vi "Floor_Negative.vi"(8 "Cutoff U8":u8, 10 "Baseline U8":u8, 11 "Input Value":u8) -> (0 "Over?":bool, 3 "Output Value":u8)   [LabVIEW 2012]
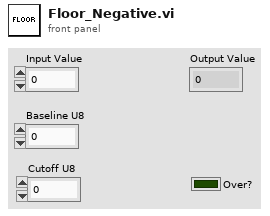
[diagram p1: front panel]
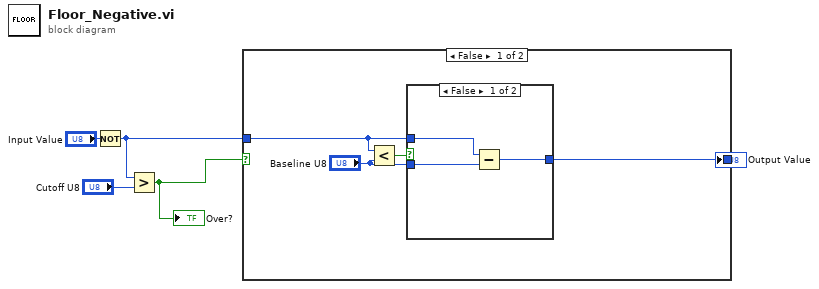
[diagram p0: block diagram]
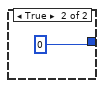
[diagram p2: hidden frame]
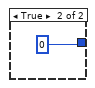
[diagram p3: hidden frame]
diagram:
  n1 = Not(x="Input Value") -> (.not. x?=w3:u8)
  n2 = Greater?(x=w3, y="Cutoff U8") -> (0:w1:bool)
  "Over?" <- w1
  n3 = case shown="False" w1 {
    tunnel: w3 -> [w8 _]
    tunnel: [w7 u8 0] -> w4
    frame False {
      n4 = Less?(x=w8, y="Baseline U8") -> (x < y?=w9:bool)
      n5 = case shown="False" w9 {
        tunnel: w8 -> [w12 _]
        tunnel: "Baseline U8" -> [w11 _]
        tunnel: [w10 u8 0] -> w7
        frame False {
          n6 = Subtract(x=w12, y=w11) -> (x-y=w10:u8)
        }
        frame True {
        }
      }
    }
    frame True {
    }
  }
  "Output Value" <- w4
